vi "Core_ClusterToByteArray.vi"(5 "Endian-ness (T, Big)":bool=TRUE, 7 "#pragma directive (0, default)":i32, 8 "error in (no error)":errorcluster, 9 "data string (big endian)":string, 10 "String Taget Alignment (1)":i32=1, 11 "type string":i16[](array[numeric])) -> (0 "error out":errorcluster, 1 "Element Sizes (used in padding calculation)":i32[](array[numeric]), 2 "Data Element Algnment Target":i32[](array[numeric]), 3 "Cluster Data as Byte Array Out":u8[](array[numeric]), 4 "Data Mask":bool[](array[boolean]), 6 "Base Data Element Info":T1[](array[typedef]))   [LabVIEW 2020]
doc: "Evaluate a cluster as a variant \"type\" and flattened string (big endian). This function uses a recursive decomposition scheme to convert each data element into a byte array (including nested clusters). \n\nWhen not wired or #pragma pack is \"0, default\" this function uses the standard C rules to insert \"padding\" in the data stream. This default may be overridden which will change the packing rules slightly. \n\nAs each element is evaluated the bytes may be reversed to accommodate target endian-ness (note, stings are not endian-dependent). \n\nAlso created is a \"Data Mask\" which is a Boolean array to signify which data bytes are \"real\" and which are padding. This mask is required to translate the data array back to a LabVIEW cluster."
uses:
  TypeDefs/ctl_DataElementInfo.ctl
panel:
  # "### BSD License (http://www.opensource.org/licenses/bsd-license.php) Begin ###\n \nCopyright (c) 2014 Jeffrey Holt <jolt.holt@gmail.com>\n\nAll rights reserved.\n\nRedistribution and use in source and binary forms, with or without modification, are permitted provided that the following conditions are met:\n\n    * Redistributions of source code must retain the above copyright notice\n\nTHIS SOFTWARE IS PROVIDED BY THE COPYRIGHT HOLDERS AND CONTRIBUTORS \"AS IS\" AND ANY EXPRESS OR IMPLIED WARRANTIES, \nINCLUDING, BUT NOT LIMITED TO, THE IMPLIED WARRANTIES OF MERCHANTABILITY AND FITNESS FOR A PARTICULAR PURPOSE ARE \nDISCLAIMED. IN NO EVENT SHALL THE COPYRIGHT OWNER OR CONTRIBUTORS BE LIABLE FOR ANY DIRECT, INDIRECT, INCIDENTAL,\n SPECIAL, EXEMPLARY, OR CONSEQUENTIAL DAMAGES (INCLUDING, BUT NOT LIMITED TO, PROCUREMENT OF SUBSTITUTE GOODS OR \nSERVICES; LOSS OF USE, DATA, OR PROFITS; OR BUSINESS INTERRUPTION) HOWEVER CAUSED AND ON ANY THEORY OF LIABILITY, \nWHETHER IN CONTRACT, STRICT LIABILITY, OR TORT (INCLUDING NEGLIGENCE OR OTHERWISE) ARISING IN ANY WAY OUT OF THE USE \nOF THIS SOFTWARE, EVEN IF ADVISED OF THE POSSIBILITY OF SUCH DAMAGE.\n\n### BSD License End ###"
  # "Parts of the underlying code was adapted from:\n\nGet Header from TD.vi\nSplit Cluster TD.vi\nParse String with TDs.vi\n\n\n\nPlease visit http://www.OpenG.org to learn about the\nOpen Source LabVIEW software movement.\n\nNOTICE -- YOU MUST LEAVE THIS NOTICE IN PLACE.  PER THE TERMS OF THE LICENSE BELOW, YOU MAY SUBLICENSE THIS SOFTWARE \nIN ANY WAY THAT DOES NOT CONFLICT WITH THIS LICENSE.\n\n### BSD License (http://www.opensource.org/licenses/bsd-license.php) Begin ###\n \nCopyright (c) 2002, Jean-Pierre Drolet <drolet_jp@hotmail.com>\nCopyright (c) 2002-2006, Jim Kring <jim@jimkring.com>\n\nAll rights reserved.\n\nRedistribution and use in source and binary forms, with or without modification, are permitted provided that the following conditions are met:\n\n    * Redistributions of source code must retain the above copyright notice, this list of conditions and the following disclaimer.\n    * Redistributions in binary form must reproduce the above copyright notice, this list of conditions and the following disclaimer in the \n       documentation and/or other materials provided with the distribution.\n    * Neither the name of SciWare, James Kring, Inc., nor the names of its contributors may be used to endorse or promote products derived \n       from this software without specific prior written permission.\n\nTHIS SOFTWARE IS PROVIDED BY THE COPYRIGHT HOLDERS AND CONTRIBUTORS \"AS IS\" AND ANY EXPRESS OR IMPLIED WARRANTIES, \nINCLUDING, BUT NOT LIMITED TO, THE IMPLIED WARRANTIES OF MERCHANTABILITY AND FITNESS FOR A PARTICULAR PURPOSE ARE \nDISCLAIMED. IN NO EVENT SHALL THE COPYRIGHT OWNER OR CONTRIBUTORS BE LIABLE FOR ANY DIRECT, INDIRECT, INCIDENTAL,\n SPECIAL, EXEMPLARY, OR CONSEQUENTIAL DAMAGES (INCLUDING, BUT NOT LIMITED TO, PROCUREMENT OF SUBSTITUTE GOODS OR \nSERVICES; LOSS OF USE, DATA, OR PROFITS; OR BUSINESS INTERRUPTION) HOWEVER CAUSED AND ON ANY THEORY OF LIABILITY, \nWHETHER IN CONTRACT, STRICT LIABILITY, OR TORT (INCLUDING NEGLIGENCE OR OTHERWISE) ARISING IN ANY WAY OUT OF THE USE \nOF THIS SOFTWARE, EVEN IF ADVISED OF THE POSSIBILITY OF SUCH DAMAGE.\n\n### BSD License End ###"
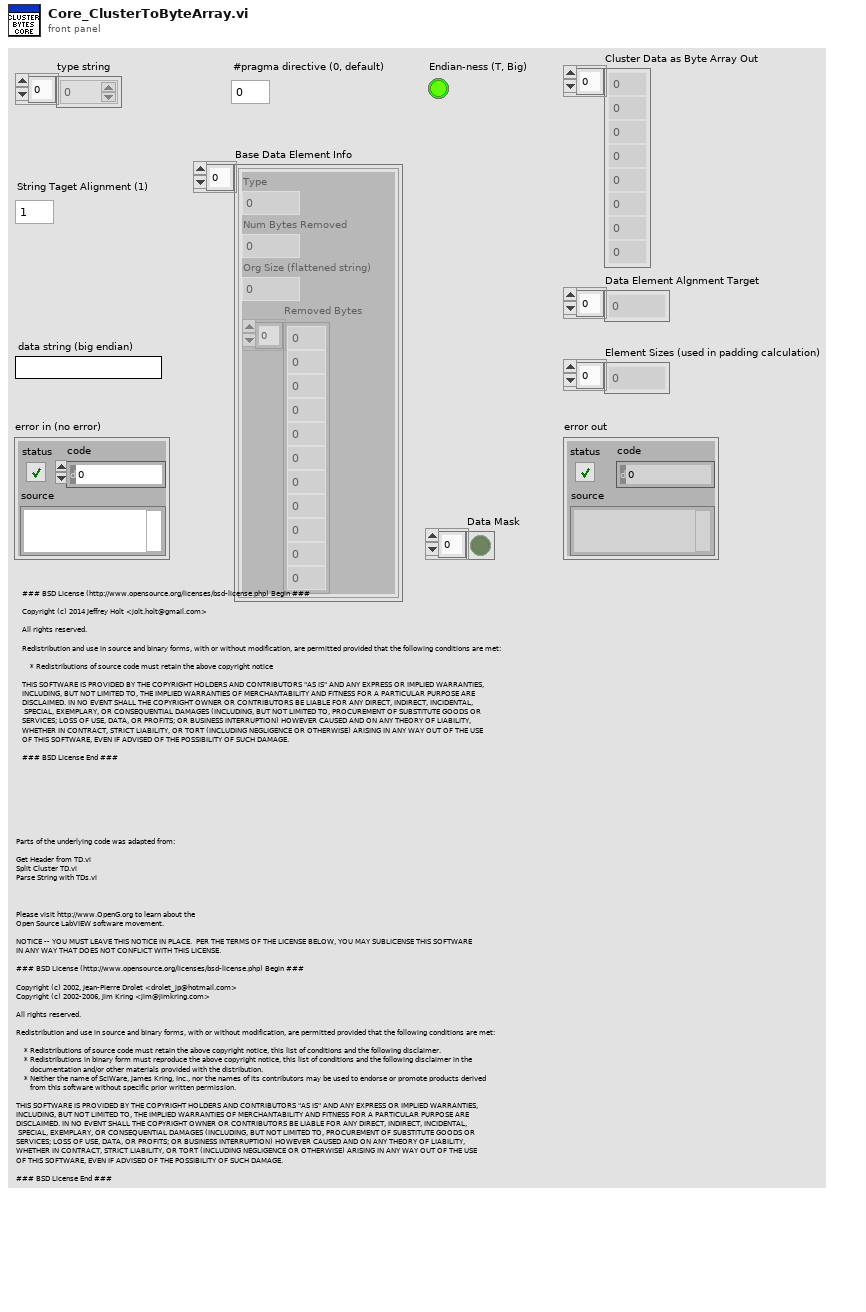
[diagram p1: front panel]
types:
  T1 = typedef "ctl_DataElementInfo.ctl" = cluster{"Type":u16, "Num Bytes Removed":u16, "Org Size (flattened string)":i32, "Removed Bytes":u8[]}
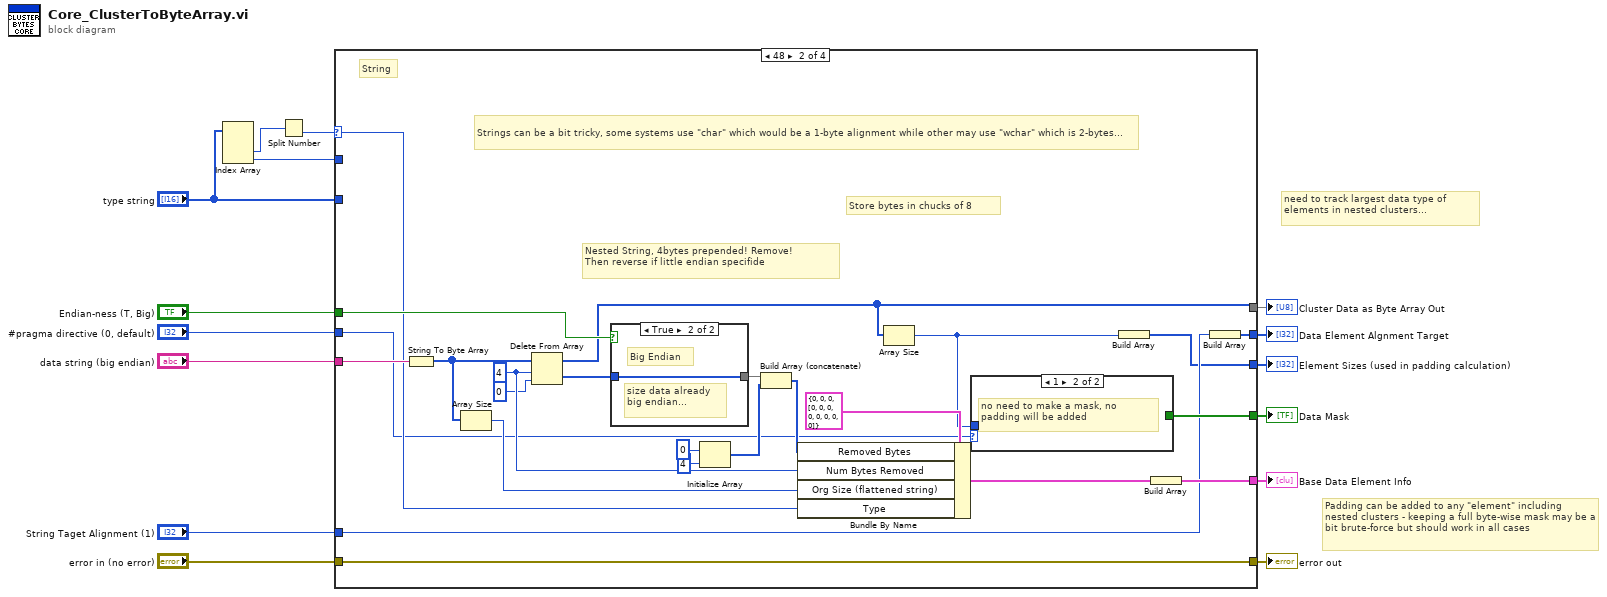
[diagram p0: block diagram]
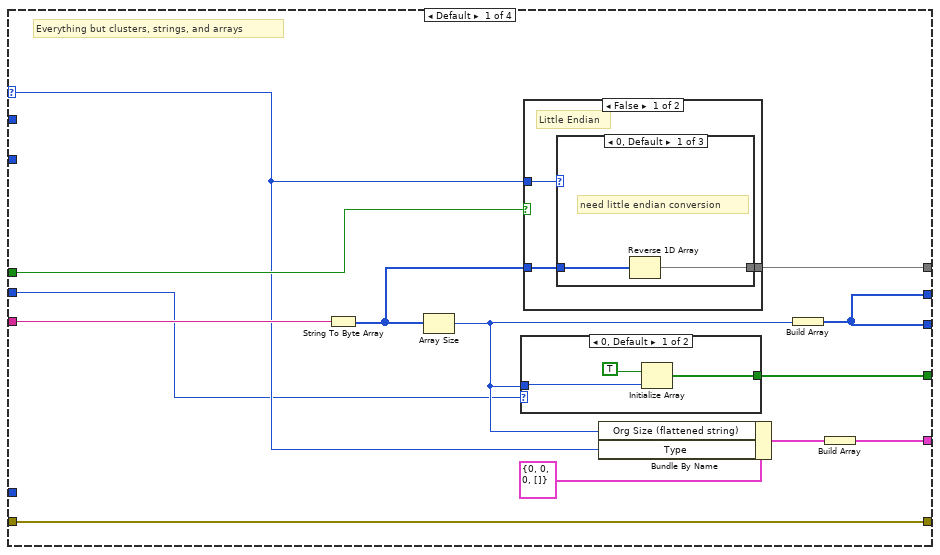
[diagram p2: hidden frame]
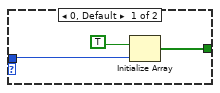
[diagram p7: hidden frame]
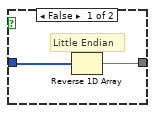
[diagram p8: hidden frame]
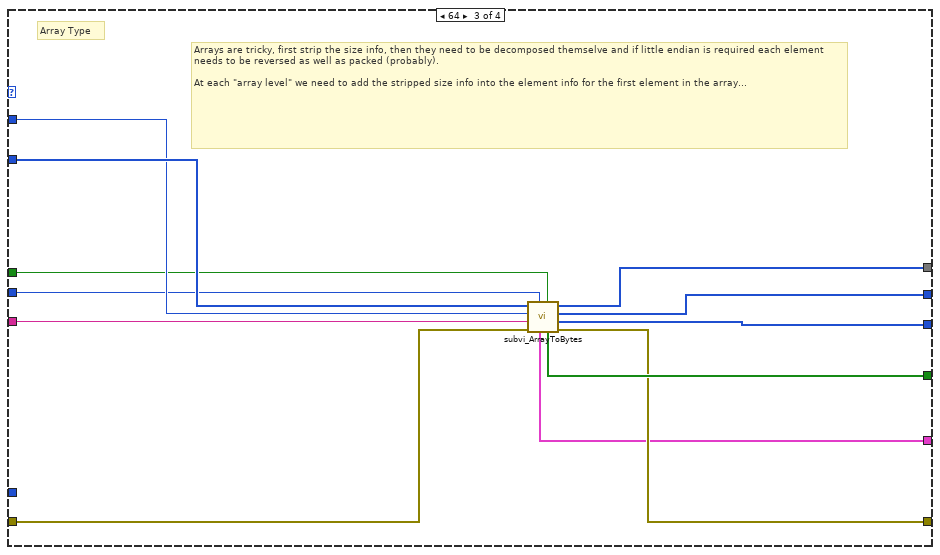
[diagram p9: hidden frame]
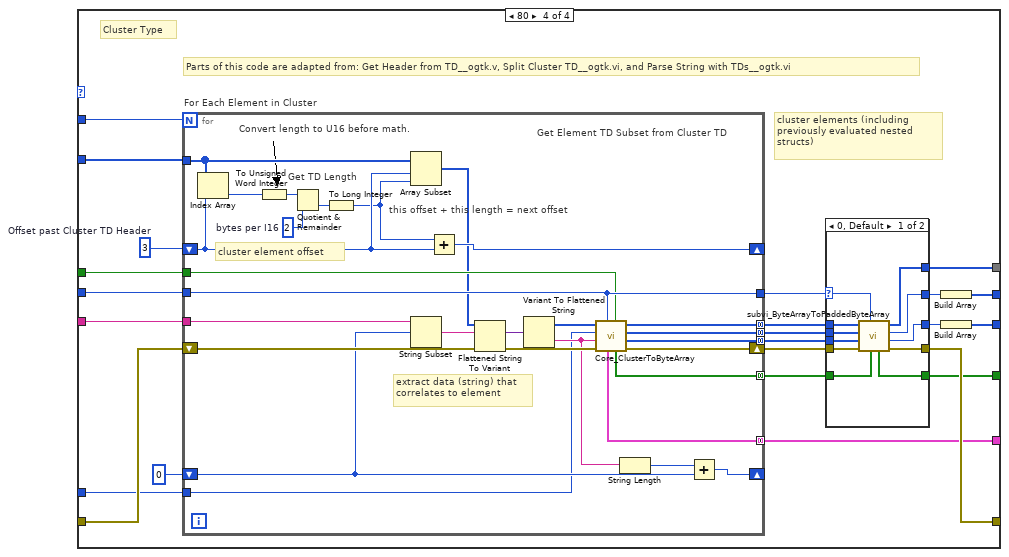
[diagram p10: hidden frame]
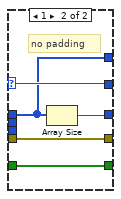
[diagram p11: hidden frame]
diagram:
  # "Padding can be added to any \"element\" including nested clusters - keeping a full byte-wise mask may be a bit brute-force but should work in all cases"
  # "need to track largest data type of elements in nested clusters..."
  n1 = Index Array(array="type string") -> (element #2=w14:i16, element #3=w13:i16)  [unwired: 3 in, 1 out]
  n2 = Split Number(x=w14) -> (lo(x)=w15:u8)  [unwired: 1 out]
  n3 = case shown="48" w15 {
    selector: w15 -> [w17 w53 _ _]
    tunnel: w13 -> [_ _ w80 w101]
    tunnel: "type string" -> [_ _ w81 w103]
    tunnel: "data string (big endian)" -> [w27 w63 w77 w102]
    tunnel: [w26 w52 w71 w91] -> w12
    tunnel: [w28 w40 w72 w99] -> w11
    tunnel: "#pragma directive (0, default)" -> [w16 w43 w79 w97]
    tunnel: "Endian-ness (T, Big)" -> [w23 w61 w78 w96]
    tunnel: [w28 w41 w73 w95] -> w8
    tunnel: "error in (no error)" -> [w25 w62 w74 w89]
    tunnel: [w25 w62 w75 w88] -> w6
    tunnel: [w24 w45 w76 w85] -> w3
    tunnel: [w20 w55 w70 w84] -> w2
    tunnel: "String Taget Alignment (1)" -> [_ w42 _ w82]
    frame Default {
      # "Everything but clusters, strings, and arrays"
      n4 = String To Byte Array(string=w27) -> (unsigned byte array=w18:u8[])
      n5 = Array Size(array=w18) -> (size(s)=w19:i32)
      n6 = case shown="0, Default" w16 {
        tunnel: [w30 _] -> w24
        tunnel: w19 -> [w29 _]
        frame 0, Default {
          n7 = Initialize Array(TRUE, w29) -> (w30:bool[])
        }
        frame 1 {
          # "no need to make a mask, no padding will be added"
        }
      }
      n8 = case shown="False" w23 {
        tunnel: [w34 w39] -> w26
        tunnel: w17 -> [w33 _]
        tunnel: w18 -> [w32 w39]
        frame False {
          # "Little Endian"
          n9 = case shown="0, Default" w33 {
            tunnel: [w36 w37 w38] -> w34
            tunnel: w32 -> [w35 w37 w38]
            frame 0, Default {
              # "need little endian conversion"
              n10 = Reverse 1D Array(array=w35) -> (reversed array=w36:u8[])
            }
            frame 48 {
              # "String, do not reverse,"
            }
            frame 50 {
              # "Path, do not reverse,"
            }
          }
        }
        frame True {
          # "Big Endian"
          # "data already big endian..."
        }
      }
      n11 = Bundle By Name(cluster=T1 {"Type"=0, "Num Bytes Removed"=0, "Org Size (flattened string)"=0, "Removed Bytes"=[]} ("Data Element Info"), "Org Size (flattened string)"=w19, "Type"=w17) -> (w21:T1)
      n12 = Build Array(w19) -> (w28:i32[])
      n13 = Build Array(w21) -> (w20:T1[])
    }
    frame 48 {
      w59 = 4 ("length")
      # "Strings can be a bit tricky, some systems use \"char\" which would be a 1-byte alignment while other may use \"wchar\" which is 2-bytes..."
      # "Store bytes in chucks of 8"
      # "Nested String, 4bytes prepended! Remove!\nThen reverse if little endian specifide"
      # "String"
      n14 = String To Byte Array(string=w63) -> (unsigned byte array=w58:u8[])
      n15 = Array Size(array=w58) -> (size(s)=w57:i32)
      n16 = Delete From Array(array=w58, length=w59, index=0) -> (deleted portion=w51:u8[], array with subset deleted=w52:u8[])
      n17 = case shown="True" w61 {
        tunnel: [w67 w69] -> w48
        tunnel: w51 -> [w68 w69]
        frame False {
          # "Little Endian"
          n18 = Reverse 1D Array(array=w68) -> (reversed array=w67:u8[])
        }
        frame True {
          # "Big Endian"
          # "size data already big endian..."
        }
      }
      n19 = Initialize Array(u8 0, 4 ("dimension size")) -> (w47:u8[])
      n20 = Build Array (concatenate)(w48, w47) -> (w46:u8[])
      n21 = Bundle By Name(cluster=T1 {"Type"=0, "Num Bytes Removed"=0, "Org Size (flattened string)"=0, "Removed Bytes"=[0, 0, 0, 0, 0, 0, 0, 0]} ("Data Element Info"), "Removed Bytes"=w46, "Num Bytes Removed"=w59, "Org Size (flattened string)"=w57, "Type"=w53) -> (w56:T1)
      n22 = Array Size(array=w52) -> (size(s)=w44:i32)
      n23 = case shown="1" w43 {
        tunnel: [w65 _] -> w45
        tunnel: w44 -> [w64 _]
        frame 0, Default {
          n24 = Initialize Array(TRUE, w64) -> (w65:bool[])
        }
        frame 1 {
          # "no need to make a mask, no padding will be added"
        }
      }
      n25 = Build Array(w44) -> (w41:i32[])
      n26 = Build Array(w56) -> (w55:T1[])
      n27 = Build Array(w42) -> (w40:i32[])
    }
    frame 64 {
      # "Array Type"
      # "Arrays are tricky, first strip the size info, then they need to be decomposed themselve and if little endian is required each element needs to be reversed as well as packed (probably).\n\nAt each \"array level\" we need to add the stripped size info into the element info for the first element in the array..."
      n28 = call "subvi_ArrayToBytes.vi"("Endian-ness (T, Big)"=w78, "#pragma directive (0, default)"=w79, "error in (no error)"=w74, "data string"=w77, "Dims \"N\""=w80, "type string"=w81) -> ("error out"=w75:errorcluster, "Element Sizes"=w73:i32[], "Data Element Algnment Target"=w72:i32[], "Cluster Data as Byte Array Out"=w71:u8[], "Data Mask"=w76:bool[], "Base Data Element Info"=w70:T1[])
    }
    frame 80 {
      w104 = 3  # Offset past Cluster TD Header
      # "Cluster Type"
      # "cluster elements (including previously evaluated nested structs)"
      # "Parts of this code are adapted from: Get Header from TD__ogtk.v, Split Cluster TD__ogtk.vi, and Parse String with TDs__ogtk.vi"
      n29 = for "For Each Element in Cluster" {
        N: w101 -> [_]
        shift-right: [w147] -> _
        shift-left: w104 -> [w146]
        tunnel: w103 -> [w148]
        tunnel: w102 -> [w139]
        shift-right: [w124] -> _
        shift-left: 0 ("Offset In") -> [w122]
        tunnel: [w138] -> w100 mode=concatenating
        tunnel: [w137] -> w98 mode=concatenating
        tunnel: w97 -> [w136]
        tunnel: w96 -> [w135]
        tunnel: [w136] -> w83
        tunnel: [w134] -> w93 mode=concatenating
        shift-right: [w133] -> w90
        shift-left: w89 -> [w131]
        tunnel: [w125] -> w86 mode=concatenating
        tunnel: [w123] -> w84 mode=concatenating
        tunnel: w82 -> [w121]
        w143 = u16 2  # bytes per I16
        # "extract data (string) that correlates to element"
        # "Get TD Length"
        # "this offset + this length = next offset"
        # "cluster element offset"
        # "Get Element TD Subset from Cluster TD"
        # "Convert length to U16 before math."
        n30 = Index Array(array=w148, index=w146) -> (element=w144:i16)
        n31 = To Unsigned Word Integer(number=w144) -> (unsigned 16bit integer=w142:u16)
        n32 = Quotient & Remainder(x=w142, y=w143) -> (floor(x/y)=w145:u16)  [unwired: 1 out]
        n33 = To Long Integer(number=w145) -> (32bit integer=w141:i32)
        n34 = Array Subset(array=w148, index=w146, length=w141) -> (w130:i16[])
        n35 = String Subset(string=w139, offset (0)=w122) -> (substring=w140:string)  [unwired: 1 in]
        n36 = Add(x=w141, y=w146) -> (x+y=w147:i32)
        n37 = Flattened String To Variant(4:w131, 6:w140, 7:w130) -> (0:w132:errorcluster, 3:w128:variant)
        n38 = Variant To Flattened String(Variant=w128) -> (data string=w127:string, 1:w126:i16[])
        n39 = call "Core_ClusterToByteArray.vi"("Endian-ness (T, Big)"=w135, "#pragma directive (0, default)"=w136, "error in (no error)"=w132, "data string (big endian)"=w127, "String Taget Alignment (1)"=w121, "type string"=w126) -> ("error out"=w133:errorcluster, "Element Sizes (used in padding calculation)"=w134:i32[], "Data Element Algnment Target"=w138:i32[], "Cluster Data as Byte Array Out"=w137:u8[], "Data Mask"=w125:bool[], "Base Data Element Info"=w123:T1[])
        n40 = String Length(string=w127) -> (length=w129:i32)
        n41 = Add(x=w129, y=w122) -> (x+y=w124:i32)
      }
      n42 = case shown="0, Default" w83 {
        selector: w83 -> [w105 w120]
        tunnel: w100 -> [w115 _]
        tunnel: w98 -> [w114 w118]
        tunnel: [w113 w119] -> w94
        tunnel: w93 -> [w112 _]
        tunnel: [w111 w120] -> w92
        tunnel: [w110 w118] -> w91
        tunnel: w90 -> [w109 w117]
        tunnel: [w108 w117] -> w88
        tunnel: w86 -> [w107 w116]
        tunnel: [w106 w116] -> w85
        frame 0, Default {
          n43 = call "subvi_ByteArrayToPaddedByteArray.vi"("Padding Mask In"=w107, "#pragma directive (0, default)"=w105, "error in (no error)"=w109, "Element Sizes"=w112, "Alignment Targets"=w115, "Cluster Data as Byte Array"=w114) -> ("error out"=w108:errorcluster, "Total Size"=w113:i32, "Alignment Target Out"=w111:i32, "Bytes Out (Padded as Needed)"=w110:u8[], "Padding Mask Out"=w106:bool[])  [unwired: 1 out]
        }
        frame 1 {
          # "no padding"
          n44 = Array Size(array=w118) -> (size(s)=w119:i32)
        }
      }
      n45 = Build Array(w92) -> (w99:i32[])
      n46 = Build Array(w94) -> (w95:i32[])
    }
  }
  "error out" <- w6
  "Cluster Data as Byte Array Out" <- w12
  "Data Element Algnment Target" <- w11
  "Element Sizes (used in padding calculation)" <- w8
  "Data Mask" <- w3
  "Base Data Element Info" <- w2
